vi "Set Error.vi"(10 "error in (no error)":errorcluster, 11 "Response in":refnum<class "Response.lvclass">) -> (3 "Response out":refnum<class "Response.lvclass">)   [LabVIEW 2022 SP3, in "obs-websocket-lv.lvlib" / "Response.lvclass"]
uses:
  Response.lvclass
  Response.lvclass/Response.ctl
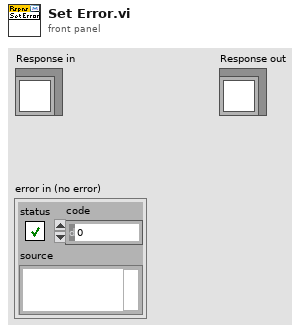
[diagram p1: front panel]
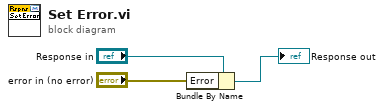
[diagram p0: block diagram]
diagram:
  n1 = Bundle By Name(cluster="Response in", "Error"="error in (no error)") -> (→"Response out":refnum<class "Response.lvclass">)
